vi "AWG Get Capabilities.vi"(8 "error in (no error)":errorcluster, 11 "awg session":T3={"type"=enum."Agilent 331xxA to 332xxA", "VISA"="", "enable 10MHz ref"=FALSE, "cmi ckd2"={"VISA"="", "clock source"=enum."Auto", "manual ref clk"=FALSE, "ref clock [Hz]"=0.0, "div mode"=enum."Set divisor directly"}, "cmi sync v3"={"VISA"="", "baud rate [bd/s]"=115200, "source"=enum."Auto", "hv range"=enum."1kV", "fsrc is fixed"=FALSE, "fsrc [Hz]"=10000000.0, "freq integ [s]"=1.0, "freq filter"=5, "trig level"=enum."TTL 5V", "chn1 mode"=enum."Source divider", "chn1 level"=enum."Positive 5V", "chn2 mode"=enum."Source divider", "chn2 level"=enum."Positive 5V", "chn2 div"=1, "chn3 mode"=enum."Chn 1 Active", "chn3 level"=enum."Positive 5V", "chn1 div entry"=enum."Calculate nearest divisor from measured fx", "chn1 dev limit [%]"=1.0, "chn1 check dev"=FALSE}, "trigger"={"source"=enum."Immediate", "level [V]"=0.0, "coupling"=enum."DC", "slope"=enum."POS"}, "HMF2500 cfg"={"Baud Rate"=9600, "Parity"=0, "Data Bits"=8, "Flow Control"=4}} {"HMF2500 cfg"."Flow Control" items=["None", "XON/XOFF", "RTS/CTS", "XON/XOFF & RTS/CTS", "DTR/DSR", "XON/XOFF & DTR/DSR"]; "HMF2500 cfg"."Data Bits" items=["7"=7, "8"=8]; "HMF2500 cfg"."Parity" items=["None", "Odd", "Even", "Mark", "Space"]; "HMF2500 cfg"."Baud Rate" items=["300"=300, "600"=600, "1200"=1200, "2400"=2400, "4800"=4800, "9600"=9600, "19200"=19200]; "cmi sync v3"."chn2 div" min=1 max=100000000 step=1; "cmi sync v3"."fsrc [Hz]" format="%_8p"}) -> (0 "error out":errorcluster, 1 "capabilities":T1, 2 "has cfg panel?":bool, 3 "awg session out":T3={"type"=enum."Agilent 331xxA to 332xxA", "VISA"="", "enable 10MHz ref"=FALSE, "cmi ckd2"={"VISA"="", "clock source"=enum."Auto", "manual ref clk"=FALSE, "ref clock [Hz]"=0.0, "div mode"=enum."Set divisor directly"}, "cmi sync v3"={"VISA"="", "baud rate [bd/s]"=115200, "source"=enum."Auto", "hv range"=enum."1kV", "fsrc is fixed"=FALSE, "fsrc [Hz]"=10000000.0, "freq integ [s]"=1.0, "freq filter"=5, "trig level"=enum."TTL 5V", "chn1 mode"=enum."Source divider", "chn1 level"=enum."Positive 5V", "chn2 mode"=enum."Source divider", "chn2 level"=enum."Positive 5V", "chn2 div"=1, "chn3 mode"=enum."Chn 1 Active", "chn3 level"=enum."Positive 5V", "chn1 div entry"=enum."Calculate nearest divisor from measured fx", "chn1 dev limit [%]"=1.0, "chn1 check dev"=FALSE}, "trigger"={"source"=enum."Immediate", "level [V]"=0.0, "coupling"=enum."DC", "slope"=enum."POS"}, "HMF2500 cfg"={"Baud Rate"=9600, "Parity"=0, "Data Bits"=8, "Flow Control"=4}} {"HMF2500 cfg"."Flow Control" items=["None", "XON/XOFF", "RTS/CTS", "XON/XOFF & RTS/CTS", "DTR/DSR", "XON/XOFF & DTR/DSR"]; "HMF2500 cfg"."Data Bits" items=["7"=7, "8"=8]; "HMF2500 cfg"."Parity" items=["None", "Odd", "Even", "Mark", "Space"]; "HMF2500 cfg"."Baud Rate" items=["300"=300, "600"=600, "1200"=1200, "2400"=2400, "4800"=4800, "9600"=9600, "19200"=19200]; "cmi sync v3"."chn2 div" min=1 max=100000000 step=1; "cmi sync v3"."fsrc [Hz]" format="%_8p"}, 4 "has ext ref?":bool)   [LabVIEW 2020, in "AWG.lvlib"]
doc: "Get selected AWG capabilities."
uses:
  AWG.lvlib
  AWG Clock Setup Mode.ctl
  AWG Capabilities.ctl
  CMI Sync V3/Configure/CMI Sync V3 Channel 1 Divisor Entry Mode.ctl
  CMI Sync V3/CMI Sync Unit V3.lvlib
  CMI Clock Divider v2/CMI ckd2 Divisor Mode.ctl
  CMI Sync V3/Configure/CMI Sync V3 Reference Clock Source.ctl
  AWG Type.ctl
  CMI Clock Divider v2/CMI ckd2 Source Mode.ctl
  CMI Clock Divider v2/CMI ckd2 Session.ctl
  AWG Session.ctl
  CMI Sync V3/Configure/CMI Sync V3 HV input Range.ctl
  CMI Sync V3/Configure/CMI Sync V3 Trigger Input Level.ctl
  CMI Sync V3/Configure/CMI Sync V3 Channel 1 Mode.ctl
  CMI Sync V3/Configure/CMI Sync V3 Channel Output Levels.ctl
  CMI Sync V3/Configure/CMI Sync V3 Channel 2 Mode.ctl
  CMI Sync V3/Configure/CMI Sync V3 Channel 3 Mode.ctl
  CMI Sync V3/CMI Sync V3 session.ctl
  externals needed for AWG/ADC Trig Mode Source.ctl
  externals needed for AWG/ADC Trig Coupling.ctl
  externals needed for AWG/ADC Trig Slope.ctl
  externals needed for AWG/ADC Trig Config.ctl
  RaS HMF2500/HMF2500 Config.ctl
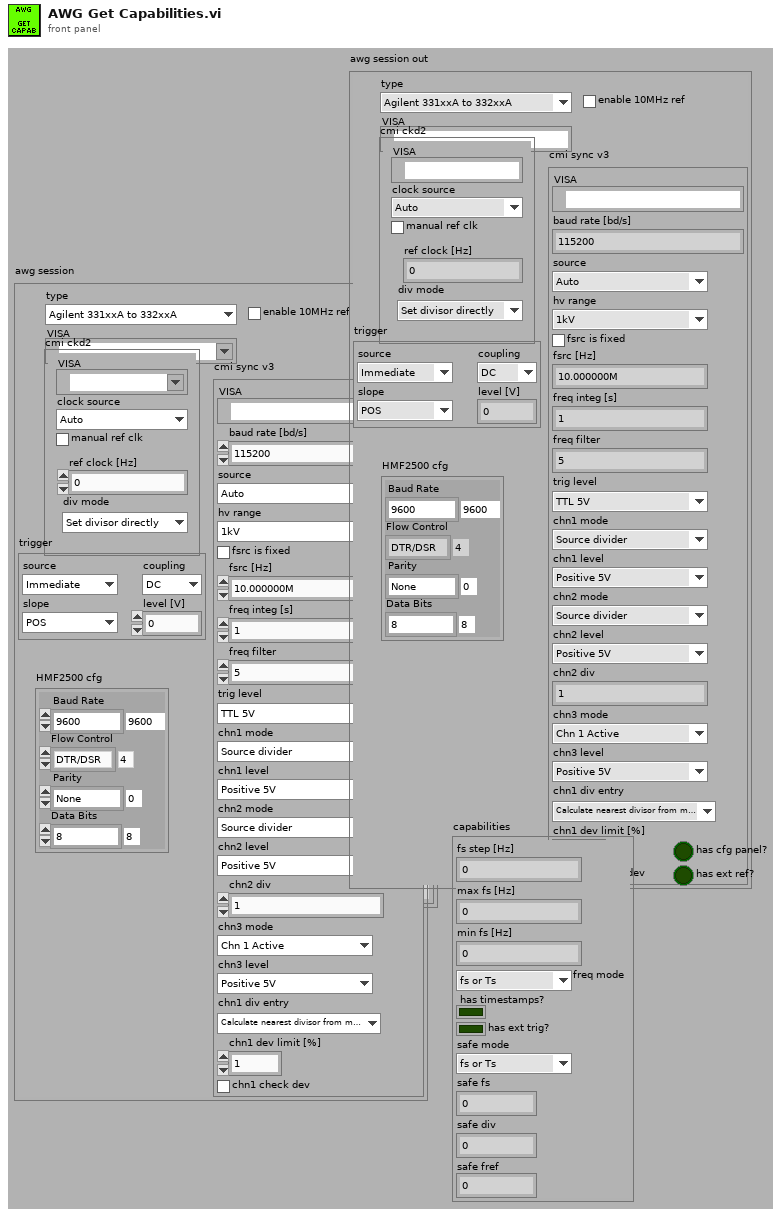
[diagram p1: front panel]
types:
  T1 = typedef "AWG.lvlib/AWG Capabilities.ctl" = cluster{"fs step [Hz]":dbl, "max fs [Hz]":dbl, "min fs [Hz]":dbl, "freq mode":T2, "has timestamps?":bool, "has ext trig?":bool, "safe mode":T2, "safe fs":dbl, "safe div":i32, "safe fref":dbl}
  T2 = typedef "AWG.lvlib/AWG Clock Setup Mode.ctl" = enum16{"fs or Ts", "fs or Ts with fref", "fref/N", "fref*M/N", "fref*Ratio"}
  T3 = typedef "AWG.lvlib/AWG Session.ctl" = cluster{"type":T4, "VISA":refnum<visa-resource-name>, "enable 10MHz ref":bool, "cmi ckd2":T5, "cmi sync v3":T8, "trigger":T17, "HMF2500 cfg":T21}
  T4 = typedef "AWG.lvlib/AWG Type.ctl" = enum16{"Agilent 331xxA to 332xxA", "Agilent 335xxA to 336xxA", "Tektronix AFG3101C", "R&S HMF25xx", "CMI Clock Divider v2", "CMI Sync Unit V3", "dummy"}
  T5 = typedef "AWG.lvlib/CMI ckd2 Session.ctl" = cluster{"VISA":refnum<visa-resource-name>, "clock source":T6, "manual ref clk":bool, "ref clock [Hz]":dbl, "div mode":T7}
  T6 = typedef "AWG.lvlib/CMI ckd2 Source Mode.ctl" = enum16{"Auto", "LF clock", "HF clock", "Internal"}
  T7 = typedef "AWG.lvlib/CMI ckd2 Divisor Mode.ctl" = enum16{"Set divisor directly", "Set divisor by frequency"}
  T8 = typedef "AWG.lvlib/CMI Sync Unit V3.lvlib/CMI Sync V3 session.ctl" = cluster{"VISA":refnum<visa-resource-name>, "baud rate [bd/s]":i32, "source":T9, "hv range":T10, "fsrc is fixed":bool, "fsrc [Hz]":dbl, "freq integ [s]":dbl, "freq filter":i32, "trig level":T11, "chn1 mode":T12, "chn1 level":T13, "chn2 mode":T14, "chn2 level":T13, "chn2 div":i32, "chn3 mode":T15, "chn3 level":T13, "chn1 div entry":T16, "chn1 dev limit [%]":dbl, "chn1 check dev":bool}
  T9 = typedef "AWG.lvlib/CMI Sync Unit V3.lvlib/CMI Sync V3 Reference Clock Source.ctl" = enum16{"Auto", "Internal", "Logic", "Sine", "HV"}
  T10 = typedef "AWG.lvlib/CMI Sync Unit V3.lvlib/CMI Sync V3 HV input Range.ctl" = enum16{"10V", "60V", "250V", "1kV"}
  T11 = typedef "AWG.lvlib/CMI Sync Unit V3.lvlib/CMI Sync V3 Trigger Input Level.ctl" = enum16{"LVCMOS 3V3", "TTL 5V"}
  T12 = typedef "AWG.lvlib/CMI Sync Unit V3.lvlib/CMI Sync V3 Channel 1 Mode.ctl" = enum16{"Source divider", "DDS absolute", "DDS ratio", "DDS ratio M/N"}
  T13 = typedef "AWG.lvlib/CMI Sync Unit V3.lvlib/CMI Sync V3 Channel Output Levels.ctl" = enum16{"Positive 3V3", "Negative 3V3", "Positive 5V", "Negative 5V"}
  T14 = typedef "AWG.lvlib/CMI Sync Unit V3.lvlib/CMI Sync V3 Channel 2 Mode.ctl" = enum16{"Source divider", "Chn 1 divide"}
  T15 = typedef "AWG.lvlib/CMI Sync Unit V3.lvlib/CMI Sync V3 Channel 3 Mode.ctl" = enum16{"Chn 1 Active", "Chn 2 Active", "Chn 1 Trigger", "Chn 2 Trigger", "Gate", "PPS", "10MHz"}
  T16 = typedef "AWG.lvlib/CMI Sync Unit V3.lvlib/CMI Sync V3 Channel 1 Divisor Entry Mode.ctl" = enum16{"Set divisor directly", "Calculate nearest divisor from measured fx"}
  T17 = typedef "ADC Trig Config.ctl" = cluster{"source":T18, "level [V]":dbl, "coupling":T19, "slope":T20}
  T18 = typedef "ADC Trig Mode Source.ctl" = enum16{"Immediate", "External", "Level"}
  T19 = typedef "ADC Trig Coupling.ctl" = enum16{"DC", "AC"}
  T20 = typedef "ADC Trig Slope.ctl" = enum16{"POS", "NEG"}
  T21 = typedef "AWG.lvlib/HMF2500 Config.ctl" = cluster{"Baud Rate":u32, "Parity":u16, "Data Bits":u16, "Flow Control":u16}
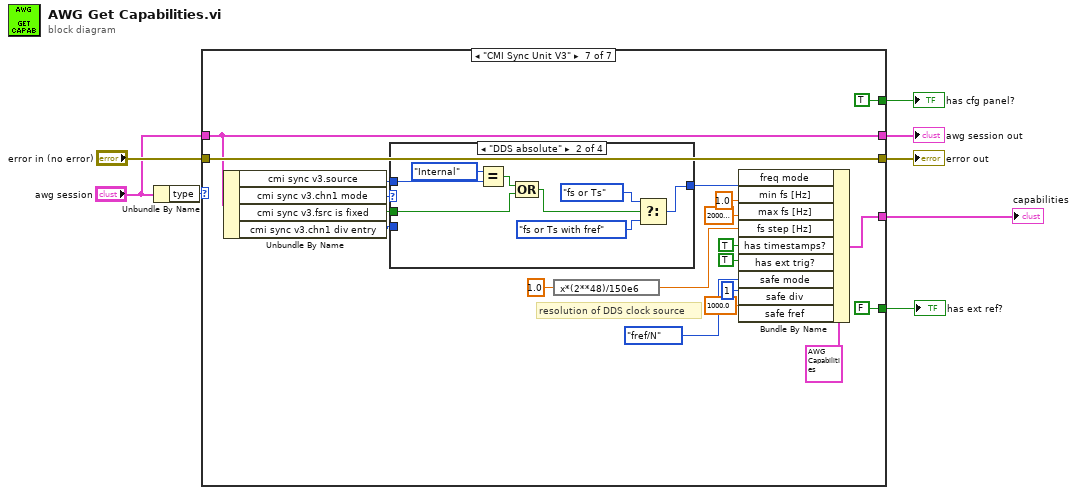
[diagram p0: block diagram]
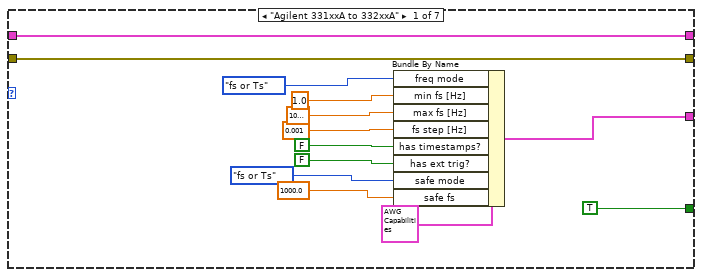
[diagram p2: hidden frame]
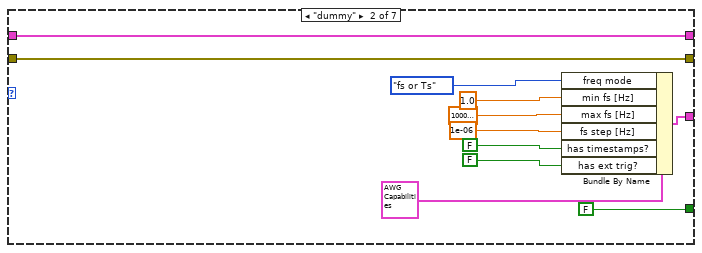
[diagram p3: hidden frame]
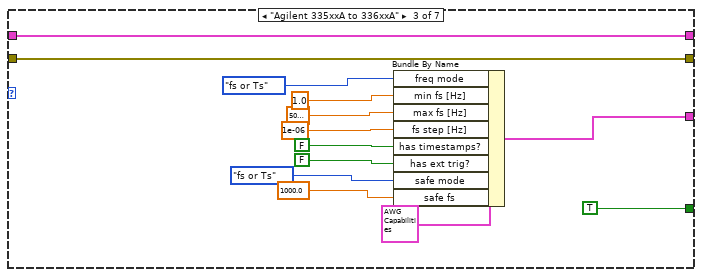
[diagram p4: hidden frame]
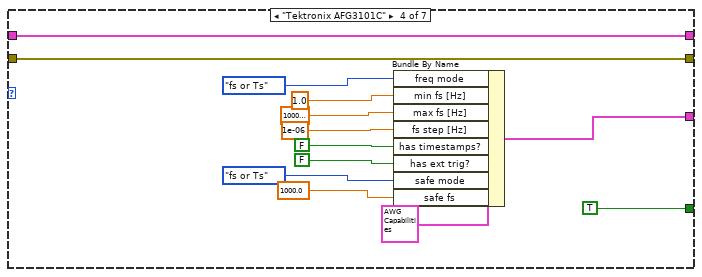
[diagram p5: hidden frame]
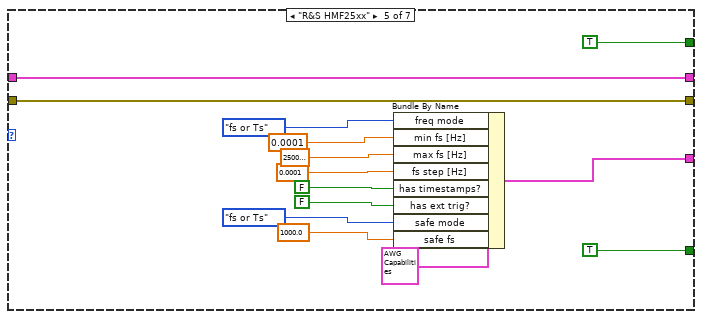
[diagram p6: hidden frame]
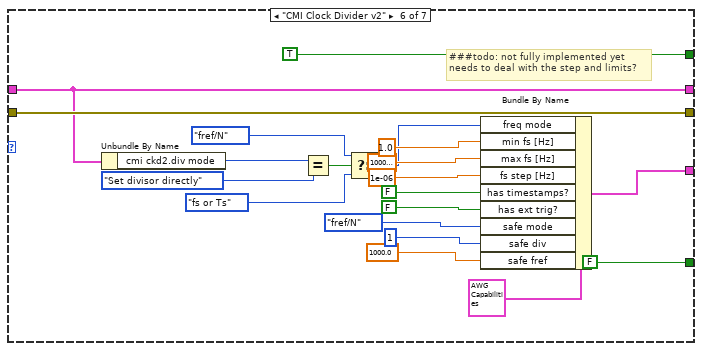
[diagram p7: hidden frame]
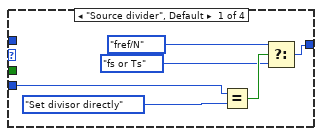
[diagram p8: hidden frame]
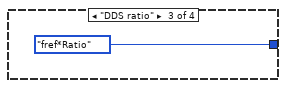
[diagram p9: hidden frame]
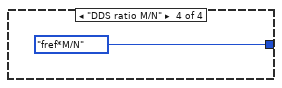
[diagram p10: hidden frame]
diagram:
  n1 = Unbundle By Name("awg session") -> ("type"=w6:T4)
  n2 = case shown="\"CMI Sync Unit V3\"" w6 {
    tunnel: "error in (no error)" -> [w20 w31 w44 w57 w71 w92 w111]
    tunnel: [w20 w31 w44 w57 w71 w92 w111] -> w7
    tunnel: "awg session" -> [w21 w32 w45 w58 w72 w83 w110]
    tunnel: [w21 w32 w45 w58 w72 w83 w110] -> w4
    tunnel: [_ _ _ _ TRUE TRUE TRUE] -> w3
    tunnel: [w13 w24 w37 w50 w64 w85 w102] -> w2
    tunnel: [TRUE FALSE TRUE TRUE TRUE FALSE FALSE] -> w1
    frame "Agilent 331xxA to 332xxA" {
      n3 = Bundle By Name(cluster=T1 {"fs step [Hz]"=0.0, "max fs [Hz]"=0.0, "min fs [Hz]"=0.0, "freq mode"=enum."fs or Ts", "has timestamps?"=FALSE, "has ext trig?"=FALSE, "safe mode"=enum."fs or Ts", "safe fs"=0.0, "safe div"=0, "safe fref"=0.0} ("capabilities"), "freq mode"=AWG_Clock_Setup_Mode."fs or Ts", "min fs [Hz]"=1.0, "max fs [Hz]"=1000000.0, "fs step [Hz]"=0.001, "has timestamps?"=FALSE, "has ext trig?"=FALSE, "safe mode"=AWG_Clock_Setup_Mode."fs or Ts", "safe fs"=1000.0) -> (w13:T1)
    }
    frame "dummy" {
      n4 = Bundle By Name(cluster=T1 {"fs step [Hz]"=0.0, "max fs [Hz]"=0.0, "min fs [Hz]"=0.0, "freq mode"=enum."fs or Ts", "has timestamps?"=FALSE, "has ext trig?"=FALSE, "safe mode"=enum."fs or Ts", "safe fs"=0.0, "safe div"=0, "safe fref"=0.0} ("capabilities"), "freq mode"=AWG_Clock_Setup_Mode."fs or Ts", "min fs [Hz]"=1.0, "max fs [Hz]"=10000000.0, "fs step [Hz]"=1e-06, "has timestamps?"=FALSE, "has ext trig?"=FALSE) -> (w24:T1)
    }
    frame "Agilent 335xxA to 336xxA" {
      n5 = Bundle By Name(cluster=T1 {"fs step [Hz]"=0.0, "max fs [Hz]"=0.0, "min fs [Hz]"=0.0, "freq mode"=enum."fs or Ts", "has timestamps?"=FALSE, "has ext trig?"=FALSE, "safe mode"=enum."fs or Ts", "safe fs"=0.0, "safe div"=0, "safe fref"=0.0} ("capabilities"), "freq mode"=AWG_Clock_Setup_Mode."fs or Ts", "min fs [Hz]"=1.0, "max fs [Hz]"=5000000.0, "fs step [Hz]"=1e-06, "has timestamps?"=FALSE, "has ext trig?"=FALSE, "safe mode"=AWG_Clock_Setup_Mode."fs or Ts", "safe fs"=1000.0) -> (w37:T1)
    }
    frame "Tektronix AFG3101C" {
      n6 = Bundle By Name(cluster=T1 {"fs step [Hz]"=0.0, "max fs [Hz]"=0.0, "min fs [Hz]"=0.0, "freq mode"=enum."fs or Ts", "has timestamps?"=FALSE, "has ext trig?"=FALSE, "safe mode"=enum."fs or Ts", "safe fs"=0.0, "safe div"=0, "safe fref"=0.0} ("capabilities"), "freq mode"=AWG_Clock_Setup_Mode."fs or Ts", "min fs [Hz]"=1.0, "max fs [Hz]"=10000000.0, "fs step [Hz]"=1e-06, "has timestamps?"=FALSE, "has ext trig?"=FALSE, "safe mode"=AWG_Clock_Setup_Mode."fs or Ts", "safe fs"=1000.0) -> (w50:T1)
    }
    frame "R&S HMF25xx" {
      n7 = Bundle By Name(cluster=T1 {"fs step [Hz]"=0.0, "max fs [Hz]"=0.0, "min fs [Hz]"=0.0, "freq mode"=enum."fs or Ts", "has timestamps?"=FALSE, "has ext trig?"=FALSE, "safe mode"=enum."fs or Ts", "safe fs"=0.0, "safe div"=0, "safe fref"=0.0} ("capabilities"), "freq mode"=AWG_Clock_Setup_Mode."fs or Ts", "min fs [Hz]"=0.0001, "max fs [Hz]"=25000000.0, "fs step [Hz]"=0.0001, "has timestamps?"=FALSE, "has ext trig?"=FALSE, "safe mode"=AWG_Clock_Setup_Mode."fs or Ts", "safe fs"=1000.0) -> (w64:T1)
    }
    frame "CMI Clock Divider v2" {
      # "###todo: not fully implemented yet\nneeds to deal with the step and limits?"
      n8 = Unbundle By Name(w83) -> ("cmi ckd2.div mode"=w82:T7)
      n9 = Equal?(x=w82, y=CMI_ckd2_Divisor_Mode."Set divisor directly") -> (x = y?=w80:bool)
      n10 = Select(t=AWG_Clock_Setup_Mode."fref/N" ("freq mode"), s=w80, f=AWG_Clock_Setup_Mode."fs or Ts" ("freq mode")) -> (s? t:f=w77:T2)
      n11 = Bundle By Name(cluster=T1 {"fs step [Hz]"=0.0, "max fs [Hz]"=0.0, "min fs [Hz]"=0.0, "freq mode"=enum."fs or Ts", "has timestamps?"=FALSE, "has ext trig?"=FALSE, "safe mode"=enum."fs or Ts", "safe fs"=0.0, "safe div"=0, "safe fref"=0.0} ("capabilities"), "freq mode"=w77, "min fs [Hz]"=1.0, "max fs [Hz]"=10000000.0, "fs step [Hz]"=1e-06, "has timestamps?"=FALSE, "has ext trig?"=FALSE, "safe mode"=AWG_Clock_Setup_Mode."fref/N", "safe div"=1, "safe fref"=1000.0) -> (w85:T1)
    }
    frame "CMI Sync Unit V3" {
      # "resolution of DDS clock source"
      n12 = Unbundle By Name(w110) -> ("cmi sync v3.source"=w93:T9, "cmi sync v3.chn1 mode"=w109:T12, "cmi sync v3.fsrc is fixed"=w108:bool, "cmi sync v3.chn1 div entry"=w98:T16)
      n13 = case shown="\"DDS absolute\"" w109 {
        tunnel: w108 -> [_ w120 _ _]
        tunnel: [w114 w126 AWG_Clock_Setup_Mode."fref*Ratio" ("freq mode") AWG_Clock_Setup_Mode."fref*M/N" ("freq mode")] -> w103
        tunnel: w98 -> [w117 _ _ _]
        tunnel: w93 -> [_ w123 _ _]
        frame "Source divider", Default {
          n14 = Equal?(x=w117, y=CMI_Sync_V3_Channel_1_Divisor_Entry_Mode."Set divisor directly" ("cmi sync v3.chn1 div entry")) -> (x = y?=w116:bool)
          n15 = Select(t=AWG_Clock_Setup_Mode."fref/N" ("freq mode"), s=w116, f=AWG_Clock_Setup_Mode."fs or Ts") -> (s? t:f=w114:T2)
        }
        frame "DDS absolute" {
          n16 = Equal?(x=CMI_Sync_V3_Reference_Clock_Source."Internal", y=w123) -> (x = y?=w121:bool)
          n17 = Compound Arithmetic op=OR(w121, w120) -> (w119:bool)
          n18 = Select(t=AWG_Clock_Setup_Mode."fs or Ts" ("freq mode"), s=w119, f=AWG_Clock_Setup_Mode."fs or Ts with fref" ("freq mode")) -> (s? t:f=w126:T2)
        }
        frame "DDS ratio" {
        }
        frame "DDS ratio M/N" {
        }
      }
      n19 = expression code="x*(2**48)/150e6"(1.0) -> (w100:dbl)
      n20 = Bundle By Name(cluster=T1 {"fs step [Hz]"=0.0, "max fs [Hz]"=0.0, "min fs [Hz]"=0.0, "freq mode"=enum."fs or Ts", "has timestamps?"=FALSE, "has ext trig?"=FALSE, "safe mode"=enum."fs or Ts", "safe fs"=0.0, "safe div"=0, "safe fref"=0.0} ("capabilities"), "freq mode"=w103, "min fs [Hz]"=1.0, "max fs [Hz]"=20000000.0, "fs step [Hz]"=w100, "has timestamps?"=TRUE, "has ext trig?"=TRUE, "safe mode"=AWG_Clock_Setup_Mode."fref/N", "safe div"=1, "safe fref"=1000.0) -> (w102:T1)
    }
  }
  "error out" <- w7
  "awg session out" <- w4
  "has cfg panel?" <- w3
  "capabilities" <- w2
  "has ext ref?" <- w1
